vi "ReferencedVariables_ReadReferencedVariable_4x4x4.vi"(8 "error in (no error)":errorcluster, 11 "reference in":refnum<class>) -> (0 "error out":errorcluster, 2 "ReplaceWithtypeDef":dbl, 3 "reference out":refnum<class>)   [LabVIEW 2010]
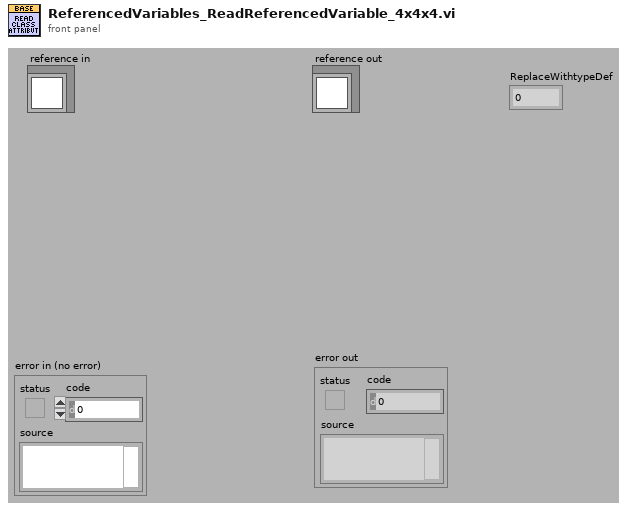
[diagram p1: front panel]
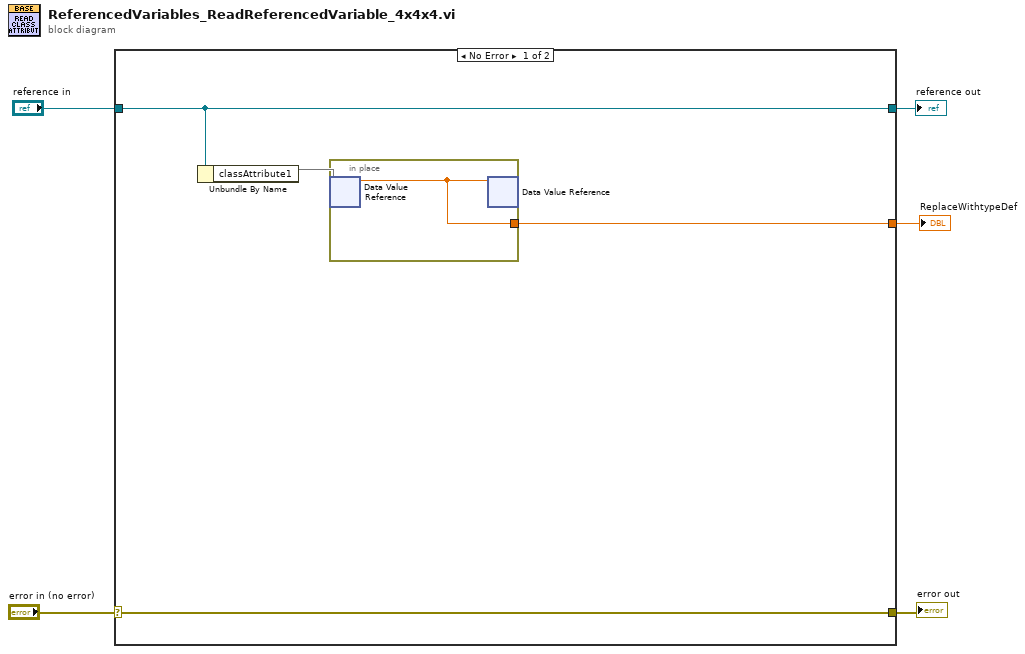
[diagram p0: block diagram]
diagram:
  n1 = case shown="No Error" "error in (no error)" {
    selector: "error in (no error)" -> [w8 w12]
    tunnel: [w8 w12] -> w4
    tunnel: [w9 w11] -> w2
    tunnel: "reference in" -> [w9 w11]
    tunnel: [w6 _] -> w1
    frame No Error {
      n2 = Unbundle By Name(w9) -> ("classAttribute1"=w7)
      n3 = in-place {
        in-place-border: [w10] -> w6
        n4 = in-place-dvr #1(w7) -> (w10:dbl)  [unwired: 1 out]
        n5 = in-place-dvr #1(w10) -> ()  [unwired: 2 out]
      }
    }
    frame Error {
    }
  }
  "error out" <- w4
  "reference out" <- w2
  "ReplaceWithtypeDef" <- w1
